vi "Magna Voltage Scan.vi"(8 "error in (no error)":errorcluster, 10 "Magna Power.lvclass":refnum<class "Magna Power.lvclass">, 11 "Magna Voltage Scan.lvclass":refnum<class "Magna Voltage Scan.lvclass">) -> (0 "error out":errorcluster, 3 "Magna Voltage Scan.lvclass 2":refnum<class "Magna Voltage Scan.lvclass">)   [LabVIEW 2017, in "Magna Voltage Scan.lvclass"]
uses:
  Magna Voltage Scan.lvclass
  C:/LabVIEW-programs-dev/Scanners/Scanner/Scanner.lvclass
  Instruments/Magna-Power Power Supply/Magna Power.lvclass
  C:/LabVIEW-programs-dev/Instruments/Utility Classes/Scannable/Scannable.lvclass
  Scanner/Scanner.lvclass
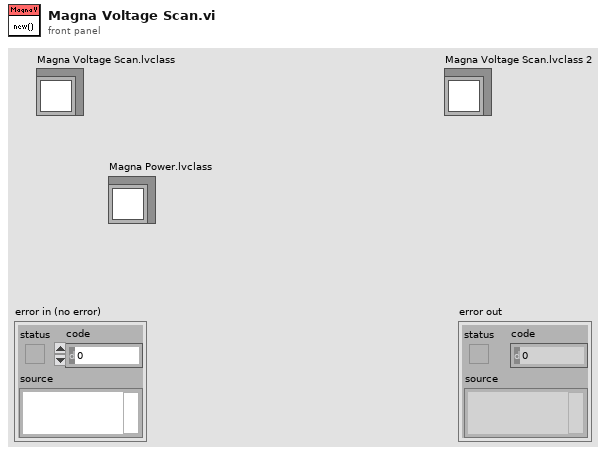
[diagram p1: front panel]
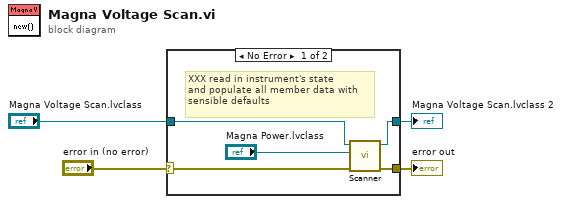
[diagram p0: block diagram]
diagram:
  n1 = case shown="No Error" "error in (no error)" {
    selector: "error in (no error)" -> [w9 w11]
    tunnel: [w8 w11] -> w3
    tunnel: [w7 w10] -> w2
    tunnel: "Magna Voltage Scan.lvclass" -> [w5 w10]
    frame No Error {
      # "XXX read in instrument's state\nand populate all member data with\nsensible defaults"
      n2 = call "Scanner.vi"("error in (no error)"=w9, "Scannable"="Magna Power.lvclass", "Scanner.lvclass in"=w5) -> ("error out"=w8:errorcluster, "Scanner.lvclass out"=w7:refnum<class "Magna Voltage Scan.lvclass">)  [unwired: 1 in, 6 out]
    }
    frame Error {
    }
  }
  "Magna Voltage Scan.lvclass 2" <- w2
  "error out" <- w3
